vi "Get Size.vi"(8 "error in (no error)":errorcluster, 11 "Proto in":refnum<class "Group.lvclass">) -> (0 "error out":errorcluster, 2 "Size":i32, 3 "Proto out":refnum<class "Group.lvclass">)   [LabVIEW 2020, in "Group.lvclass"]
uses:
  Group.lvclass
  Group.lvclass/Group.ctl
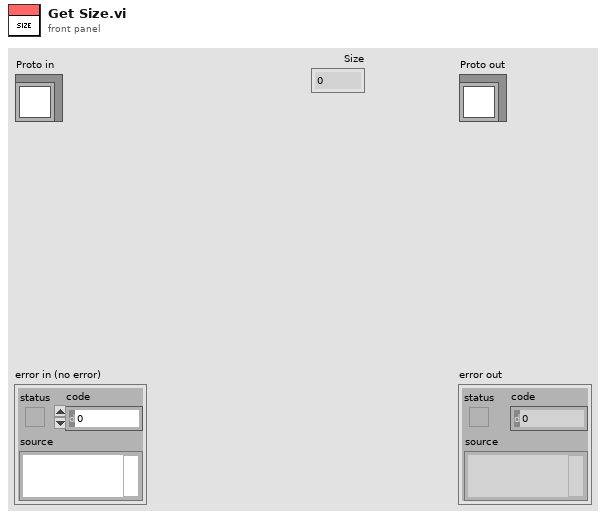
[diagram p1: front panel]
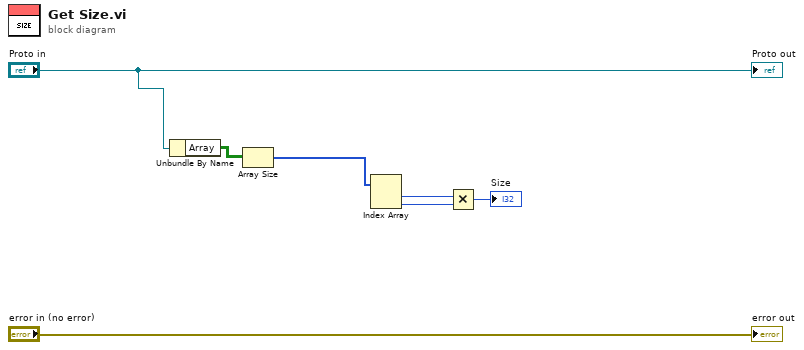
[diagram p0: block diagram]
diagram:
  n1 = Unbundle By Name("Proto in") -> ("Array"=w5:bool[][])
  n2 = Array Size(array=w5) -> (size(s)=w4:i32[])
  n3 = Index Array(array=w4) -> (element #1=w3:i32, element #2=w2:i32)  [unwired: 2 in]
  n4 = Multiply(x=w3, y=w2) -> (x*y=→"Size":i32)
  "error out" <- "error in (no error)"
  "Proto out" <- "Proto in"
